vi "flash_lamp (SubVI).vi"(8 "Flash lamp\n settings:":T1={"Flash lamp?"=FALSE, "Number of cyles\nbetween flashes"=3, "# Pulses"=35, "Stop flashing \nbelow thresh?"=FALSE, "Stop threshold"=0.001, "Pulse voltage?"=FALSE, "Pulse length (ms)"=0.001, "Pulse amp (V)"=0.001}, 9 "# Pulses in":i32, 11 "Output channel (for flashing)":tag) -> ()   [LabVIEW 2014]
uses:
  <vilib>/DAQmx/create/channels.llb/DAQmx Create Channel (AO-Voltage-Basic).vi
  <vilib>/DAQmx/configure/timing.llb/DAQmx Timing (Sample Clock).vi
  <vilib>/DAQmx/write.llb/DAQmx Write (Analog 2D DBL NChan NSamp).vi
  <vilib>/DAQmx/write.llb/DAQmx Write (Analog 1D DBL 1Chan NSamp).vi
panel:
  out "Waveform Graph":dbl[](graph)
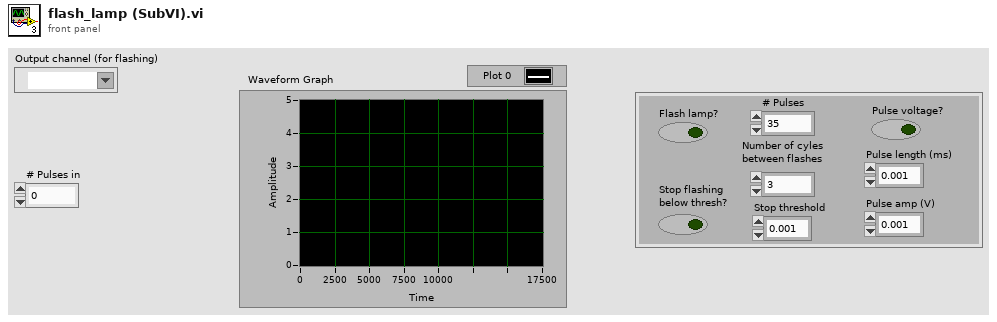
[diagram p1: front panel]
types:
  T1 = cluster{"Flash lamp?":bool, "Number of cyles\nbetween flashes":i32, "# Pulses":i32, "Stop flashing \nbelow thresh?":bool, "Stop threshold":dbl, "Pulse voltage?":bool, "Pulse length (ms)":dbl, "Pulse amp (V)":dbl}
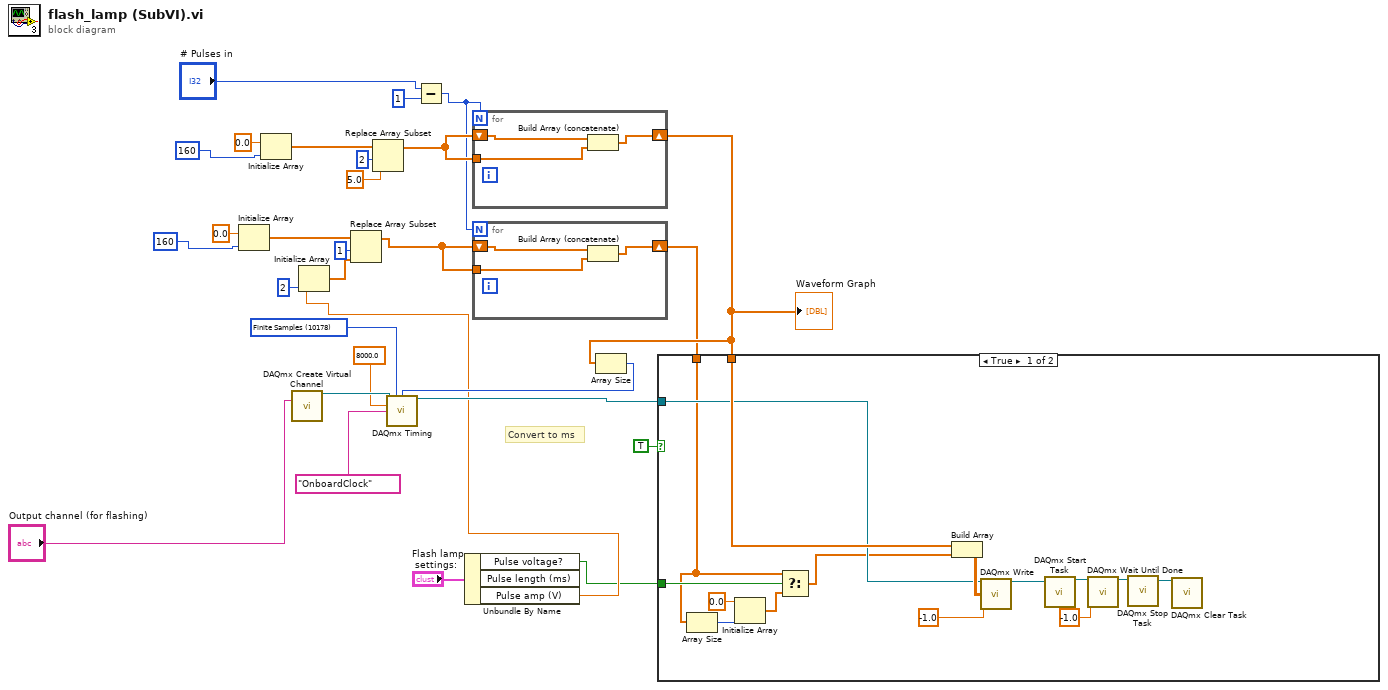
[diagram p0: block diagram]
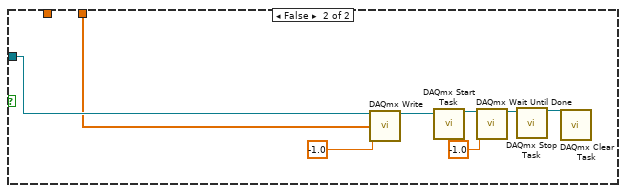
[diagram p2: hidden frame]
diagram:
  w20 = 10178 items=["Finite Samples"=10178, "Continuous Samples"=10123, "Hardware Timed Single Point"=12522] ("sample mode")
  # "Convert to ms"
  n1 = Initialize Array(0.0 ("element"), 160 ("y")) -> (w9:dbl[])
  n2 = Initialize Array(0.0 ("element"), 160 ("y")) -> (w13:dbl[])
  n3 = call-poly <vilib>:"DAQmx Create Virtual Channel.vi"("physical channels"="Output channel (for flashing)") -> ("task out"=w28:refnum<k21>)  [unwired: 13 in, 1 out]
  n4 = Replace Array Subset(array=w13, new element=5.0 ("new element/subarray"), index=2) -> (w22:dbl[])
  n5 = Subtract(x="# Pulses in", y=1) -> (x-y=w6:i32)
  n6 = Unbundle By Name("Flash lamp\n settings:") -> ("Pulse voltage?"=w1:bool, "Pulse amp (V)"=w3:dbl)  [unwired: 1 out]
  n7 = Initialize Array(w3, 2 ("dimension size")) -> (w5:dbl[])
  n8 = Replace Array Subset(array=w9, new element=w5, index=1) -> (w8:dbl[])
  n9 = for {
    N: w6 -> [_]
    shift-right: [w30] -> w14
    shift-left: w22 -> [w32]
    tunnel: w22 -> [w31]
    n10 = Build Array (concatenate)(w32, w31) -> (w30:dbl[])
  }
  "Waveform Graph" <- w14
  n11 = for {
    N: w6 -> [_]
    shift-right: [w33] -> w7
    shift-left: w8 -> [w35]
    tunnel: w8 -> [w34]
    n12 = Build Array (concatenate)(w35, w34) -> (w33:dbl[])
  }
  n13 = Array Size(array=w14) -> (size(s)=w19:i32)
  n14 = call-poly <vilib>:"DAQmx Timing.vi"("task/channels in"=w28, "sample mode"=w20, "samples per channel"=w19, "rate"=8000.0 ("Sample Rate"), "source"=tag "OnboardClock") -> ("task out"=w26:refnum<k21>)  [unwired: 9 in, 1 out]
  n15 = case shown="True" TRUE {
    tunnel: w26 -> [w42 w52]
    tunnel: w14 -> [w43 w51]
    tunnel: w7 -> [w39 _]
    tunnel: w1 -> [w41 _]
    frame True {
      n16 = Array Size(array=w39) -> (size(s)=w38:i32)
      n17 = Initialize Array(0.0 ("element"), w38) -> (w36:dbl[])
      n18 = Select(t=w39, s=w41, f=w36) -> (s? t:f=w40:dbl[])
      n19 = Build Array(w43, w40) -> (w44:dbl[][])
      n20 = call-poly <vilib>:"DAQmx Write.vi"("task/channels in"=w42, "data"=w44, "timeout"=-1.0) -> ("task out"=w49:refnum<k21>)  [unwired: 10 in, 2 out]
      n21 = call <vilib>:"DAQmx Start Task.vi"("task/channels in"=w49) -> ("task out"=w48:refnum<k21>)  [unwired: 13 in, 1 out]
      n22 = call <vilib>:"DAQmx Wait Until Done.vi"("task/channels in"=w48, "timeout (sec)"=-1.0) -> ("task out"=w47:refnum<k21>)  [unwired: 12 in, 1 out]
      n23 = call <vilib>:"DAQmx Stop Task.vi"("task/channels in"=w47) -> ("task out"=w50:refnum<k21>)  [unwired: 13 in, 1 out]
      n24 = call <vilib>:"DAQmx Clear Task.vi"("task in"=w50) -> ()  [unwired: 14 in, 1 out]
    }
    frame False {
      n25 = call-poly <vilib>:"DAQmx Write.vi"("task/channels in"=w52, "data"=w51, "timeout"=-1.0) -> ("task out"=w57:refnum<k21>)  [unwired: 10 in, 2 out]
      n26 = call <vilib>:"DAQmx Start Task.vi"("task/channels in"=w57) -> ("task out"=w56:refnum<k21>)  [unwired: 13 in, 1 out]
      n27 = call <vilib>:"DAQmx Wait Until Done.vi"("task/channels in"=w56, "timeout (sec)"=-1.0) -> ("task out"=w55:refnum<k21>)  [unwired: 12 in, 1 out]
      n28 = call <vilib>:"DAQmx Stop Task.vi"("task/channels in"=w55) -> ("task out"=w58:refnum<k21>)  [unwired: 13 in, 1 out]
      n29 = call <vilib>:"DAQmx Clear Task.vi"("task in"=w58) -> ()  [unwired: 14 in, 1 out]
    }
  }
